vi "Save-As-Default (SubVI).vi"(0 "Current VI's Path":path, 5 "Load Settings":bool, 7 "Save Settings":bool, 9 "Save and Exit":bool, 11 "Error IN":errorcluster) -> (15 "Save as Default Error":errorcluster)   [LabVIEW 2012]
panel:
  # "Save As Defaults (SubVI) - Created by Blake Otting - October 2007\nUpdated 6/26/2013"
  # "Connect As Shown \nin Main Program VI"
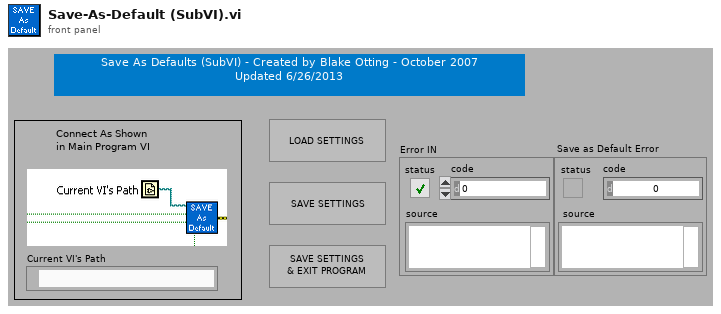
[diagram p1: front panel]
types:
  T1 = enum16{"open", "replace", "create", "open or create", "replace or create", "replace or create with confirmation"}
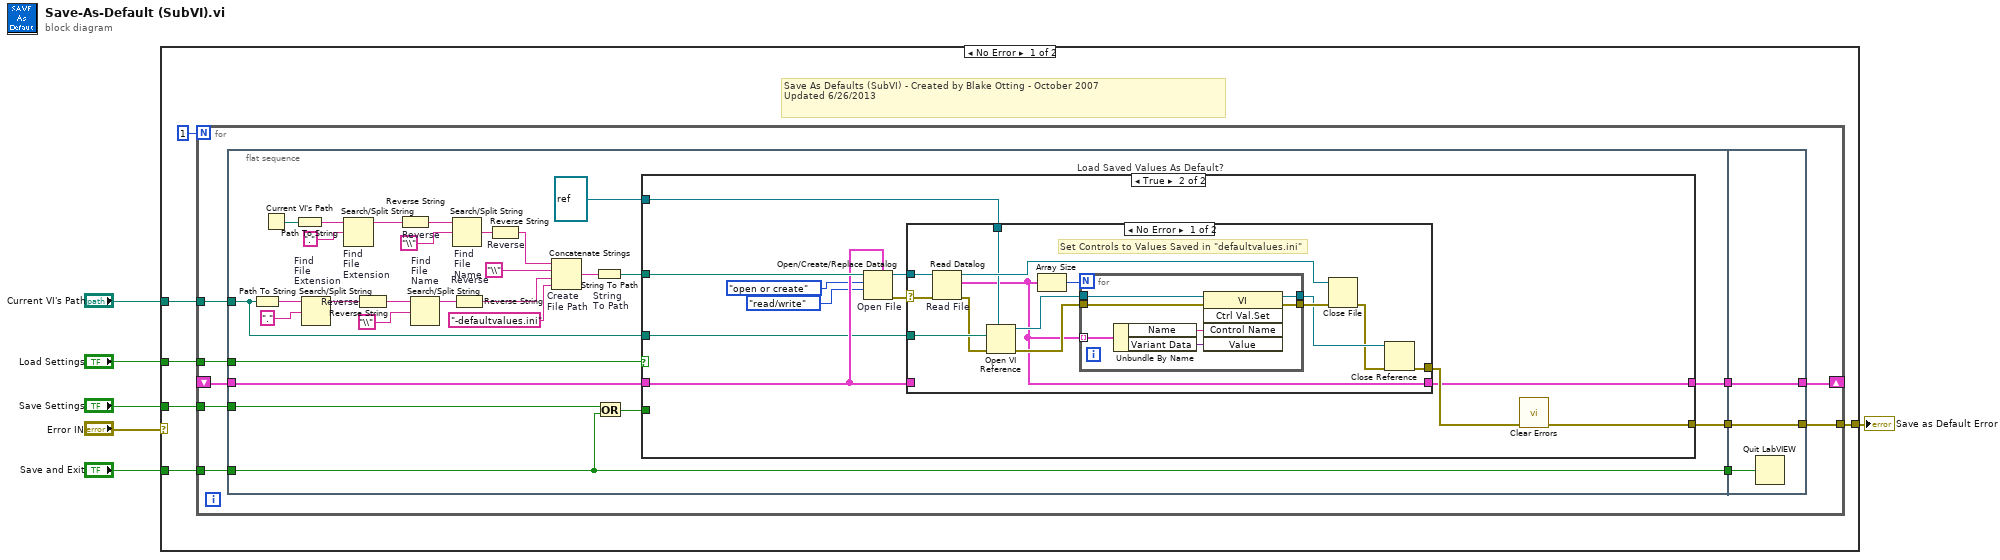
[diagram p0: block diagram]
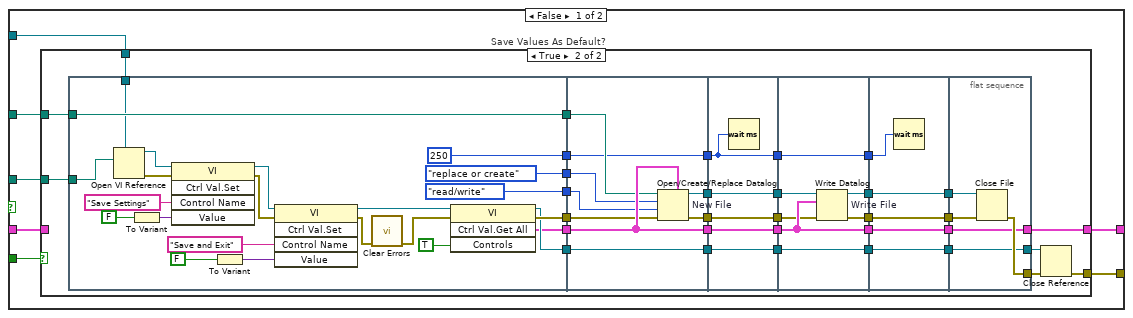
[diagram p2: hidden frame]
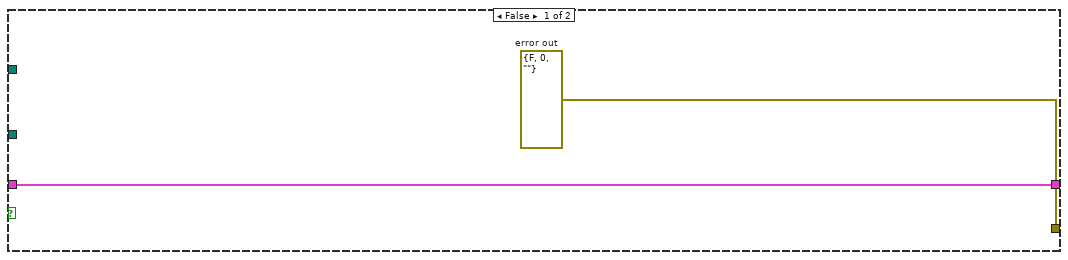
[diagram p3: hidden frame]
diagram:
  n1 = case shown="No Error" "Error IN" {
    selector: "Error IN" -> [_ w184]
    tunnel: "Save Settings" -> [w12 _]
    tunnel: "Load Settings" -> [w11 _]
    tunnel: "Save and Exit" -> [w10 _]
    tunnel: "Current VI's Path" -> [w8 _]
    tunnel: [w7 w184] -> w2
    frame No Error {
      # "Save As Defaults (SubVI) - Created by Blake Otting - October 2007\nUpdated 6/26/2013"
      n2 = for {
        N: 1 -> [_]
        tunnel: w8 -> [w21]
        shift-right: [w22] -> _
        shift-left: _ -> [w20]
        tunnel: [w19] -> w7
        tunnel: w10 -> [w14]
        tunnel: w11 -> [w13]
        tunnel: w12 -> [w15]
        n3 = flat-sequence {
          tunnel: [w49] -> w18
          tunnel: [w47] -> w17
          tunnel: [w46] -> w16
          tunnel: w13 -> [w23]
          tunnel: w14 -> [w46]
          tunnel: w15 -> [w45]
          tunnel: w21 -> [w44]
          tunnel: w20 -> [w50]
          tunnel: [w182] -> w19
          tunnel: [w183] -> w22
          tunnel: w18 -> [w183]
          tunnel: w17 -> [w182]
          tunnel: w16 -> [w181]
          frame #0 {
            n4 = Path To String(path=w44) -> (string=w32:string)
            n5 = Current VI's Path() -> (path=w27:path)
            n6 = Path To String(path=w27) -> (string=w39:string)
            n7 = Search/Split String "Find\nFile \nExtension"(string=w32, search string/char (-)=".") -> (substring before match=w29:string)  [unwired: 1 in, 2 out]
            n8 = Search/Split String "Find\nFile \nExtension"(string=w39, search string/char (-)=".") -> (substring before match=w38:string)  [unwired: 1 in, 2 out]
            n9 = Reverse String "Reverse"(1:w29) -> (0:w31:string)
            n10 = Reverse String "Reverse"(1:w38) -> (0:w37:string)
            n11 = Search/Split String "Find\nFile \nName"(string=w31, search string/char (-)="\\") -> (substring before match=w28:string)  [unwired: 1 in, 2 out]
            n12 = Search/Split String "Find\nFile \nName"(string=w37, search string/char (-)="\\") -> (match + rest of string=w35:string)  [unwired: 1 in, 2 out]
            n13 = Reverse String "Reverse"(1:w28) -> (0:w25:string)
            n14 = Reverse String "Reverse"(1:w35) -> (0:w34:string)
            n15 = Concatenate Strings "Create\nFile Path"(w34, "\\", w25, "-defaultvalues.ini") -> (w42:string)
            n16 = String To Path "String\nTo Path"(string=w42) -> (path=w43:path)
            n17 = Or(x=w45, y=w46) -> (x .or. y?=w48:bool)
            n18 = case "Load Saved Values As Default?" shown="True" w23 {
              tunnel: [w57 w147] -> w47
              tunnel: w43 -> [w56 w155]
              tunnel: w48 -> [w55 _]
              tunnel: w50 -> [w54 w154]
              tunnel: [w51 w156] -> w49
              tunnel: w44 -> [w53 w152]
              tunnel: refnum<vi> refnum ("Application Reference Input 2") -> [w52 w153]
              frame False {
                n19 = case "Save Values As Default?" shown="True" w55 {
                  tunnel: [w58 w92] -> w57
                  tunnel: w56 -> [_ w91]
                  tunnel: [w59 w90] -> w51
                  tunnel: w54 -> [w59 _]
                  tunnel: w53 -> [_ w60]
                  tunnel: w52 -> [_ w61]
                  frame False {
                    w58 = errorcluster {"status"=FALSE, "code"=0, "source"=""}  # error out
                  }
                  frame True {
                    n20 = flat-sequence {
                      tunnel: w91 -> [w115]
                      tunnel: [w97] -> w70
                      tunnel: [enum16{"read/write", "read-only", "write-only"}."read/write" ("access (0:read/write)")] -> w69
                      tunnel: [T1."replace or create" ("operation (0:open)")] -> w68
                      tunnel: [w95] -> w67
                      tunnel: [w115] -> w66
                      tunnel: [w96] -> w65
                      tunnel: [u32 250 ("milliseconds to wait")] -> w64
                      tunnel: w61 -> [w99]
                      tunnel: w60 -> [w98]
                      tunnel: [w120] -> w89
                      tunnel: [w119] -> w87
                      tunnel: [w124] -> w85
                      tunnel: [w117] -> w83
                      tunnel: [w116] -> w71
                      tunnel: w70 -> [w123]
                      tunnel: w69 -> [w122]
                      tunnel: w68 -> [w121]
                      tunnel: w67 -> [w124]
                      tunnel: w66 -> [w118]
                      tunnel: w65 -> [w117]
                      tunnel: w64 -> [w116]
                      tunnel: w89 -> [w129]
                      tunnel: [w129] -> w88
                      tunnel: w87 -> [w128]
                      tunnel: [w128] -> w86
                      tunnel: w85 -> [w127]
                      tunnel: [w127] -> w84
                      tunnel: w83 -> [w126]
                      tunnel: [w126] -> w82
                      tunnel: w71 -> [w125]
                      tunnel: [w125] -> w62
                      tunnel: w88 -> [w134]
                      tunnel: w86 -> [w136]
                      tunnel: w84 -> [w135]
                      tunnel: [w135] -> w81
                      tunnel: w82 -> [w133]
                      tunnel: [w133] -> w79
                      tunnel: [w132] -> w77
                      tunnel: [w131] -> w75
                      tunnel: [w130] -> w63
                      tunnel: w62 -> [w130]
                      tunnel: w81 -> [w141]
                      tunnel: [w141] -> w80
                      tunnel: w79 -> [w140]
                      tunnel: [w140] -> w78
                      tunnel: w77 -> [w139]
                      tunnel: [w139] -> w76
                      tunnel: w75 -> [w138]
                      tunnel: [w138] -> w74
                      tunnel: w63 -> [w137]
                      tunnel: [w145] -> w90
                      tunnel: w80 -> [w145]
                      tunnel: [w144] -> w72
                      tunnel: w78 -> [w144]
                      tunnel: w76 -> [w143]
                      tunnel: w74 -> [w142]
                      tunnel: [w146] -> w73
                      frame #0 {
                        n21 = Open VI Reference(type specifier VI Refnum (for type only)=w99, vi path=w98) -> (vi reference=w107:refnum<vi>, error out=w108:errorcluster)  [unwired: 2 in, 2 out]
                        n22 = To Variant(anything=FALSE ("Controls")) -> (Variant=w106:variant)
                        n23 = invoke class="VI" method="Ctrl Val.Set"(reference=w107, error in=w108, "Control Name"="Save Settings", "Value"=w106) -> (reference out=w111:refnum<vi>, error out=w112:errorcluster)  [unwired: 1 in, 3 out]
                        n24 = To Variant(anything=FALSE ("Controls")) -> (Variant=w109:variant)
                        n25 = invoke class="VI" method="Ctrl Val.Set"(reference=w111, error in=w112, "Control Name"="Save and Exit", "Value"=w109) -> (reference out=w114:refnum<vi>, error out=w94:errorcluster)  [unwired: 1 in, 3 out]
                        n26 = call <vilib>:"Clear Errors.vi"("error in (no error)"=w94) -> ("error out"=w93:errorcluster)  [unwired: 6 out]
                        n27 = invoke class="VI" method="Ctrl Val.Get All"(reference=w114, error in=w93, "Controls"=TRUE) -> (reference out=w96:refnum<vi>, error out=w97:errorcluster, "Get All Control Values Variant"=w95:cluster{"Name":string, "Variant Data":variant}[])  [unwired: 1 in, 1 out]
                      }
                      frame #1 {
                        n28 = Open/Create/Replace Datalog "New File"(5:w124, 8:w123, 9:w122, 10:w121, 11:w118) -> (0:w120:errorcluster, 3:w119:refnum<k1>)  [unwired: 2 out]
                      }
                      frame #2 {
                        n29 = Wait (ms)(milliseconds to wait=w125) -> ()  [unwired: 1 out]
                      }
                      frame #3 {
                        n30 = Write Datalog "Write File"(4:w134, 6:w135, 7:w136) -> (0:w132:errorcluster, 3:w131:refnum<k1>)
                      }
                      frame #4 {
                        n31 = Wait (ms)(milliseconds to wait=w137) -> ()  [unwired: 1 out]
                      }
                      frame #5 {
                        n32 = Close File(refnum=w142, error in=w143) -> (error out=w146:errorcluster)  [unwired: 1 out]
                      }
                    }
                    n33 = Close Reference(reference=w72, error in (no error)=w73) -> (error out=w92:errorcluster)
                  }
                }
              }
              frame True {
                n34 = Open/Create/Replace Datalog "Open File"(5:w154, 9:enum16{"read/write", "read-only", "write-only"}."read/write" ("access (0:read/write)"), 10:T1."open or create" ("operation (0:open)"), 11:w155) -> (0:w151:errorcluster, 3:w150:refnum<k1>)  [unwired: 1 in, 2 out]
                n35 = case shown="No Error" w151 {
                  selector: w151 -> [w166 w179]
                  tunnel: [w169 w179] -> w157
                  tunnel: w154 -> [_ w180]
                  tunnel: [w160 w180] -> w156
                  tunnel: w150 -> [w159 _]
                  tunnel: w153 -> [w164 _]
                  tunnel: w152 -> [w163 _]
                  frame No Error {
                    # "Set Controls to Values Saved in \"defaultvalues.ini\""
                    n36 = Read Datalog "Read File"(4:w166, 7:w159) -> (0:w158:errorcluster, 2:w160:cluster{"Name":string, "Variant Data":variant}[], 3:w171:refnum<k1>)  [unwired: 1 out]
                    n37 = Open VI Reference(type specifier VI Refnum (for type only)=w164, vi path=w163, error in (no error)=w158) -> (vi reference=w165:refnum<vi>, error out=w162:errorcluster)  [unwired: 1 in, 2 out]
                    n38 = Array Size(array=w160) -> (size(s)=w161:i32)
                    n39 = for {
                      N: w161 -> [_]
                      tunnel: w160 -> [w174] mode=indexing
                      tunnel: w162 -> [w176]
                      tunnel: [w177] -> w170
                      tunnel: w165 -> [w175]
                      tunnel: [w172] -> w168
                      n40 = Unbundle By Name(w174) -> ("Name"=w173:string, "Variant Data"=w178:variant)
                      n41 = invoke class="VI" method="Ctrl Val.Set"(reference=w175, error in=w176, "Control Name"=w173, "Value"=w178) -> (reference out=w172:refnum<vi>, error out=w177:errorcluster)  [unwired: 1 in, 3 out]
                    }
                    n42 = Close File(refnum=w171, error in=w170) -> (error out=w167:errorcluster)  [unwired: 1 out]
                    n43 = Close Reference(reference=w168, error in (no error)=w167) -> (error out=w169:errorcluster)
                  }
                  frame Error {
                    # "\"defaultvalues.ini\" Not Found"
                  }
                }
                n44 = call <vilib>:"Clear Errors.vi"("error in (no error)"=w157) -> ("error out"=w147:errorcluster)  [unwired: 6 in]
              }
            }
          }
          frame #1 {
            n45 = Quit LabVIEW(quit? (T)=w181) -> ()
          }
        }
      }
    }
    frame Error {
    }
  }
  "Save as Default Error" <- w2
